vi "XY Plots from Image.vi"(10 "wavelengths":dbl[](array[numeric]), 11 "Image ROI1":u16[][](array[numeric])) -> (3 "Array":T1(array[cluster]))   [LabVIEW 2019, in "Dashboard.lvlib"]
uses:
  Dashboard.lvlib
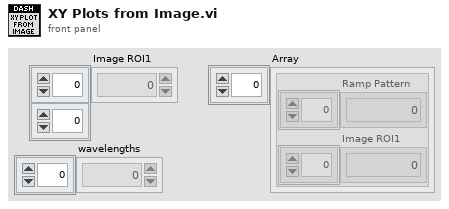
[diagram p1: front panel]
types:
  T1 = cluster{"Ramp Pattern":dbl[], "Image ROI1":u16[]}[]
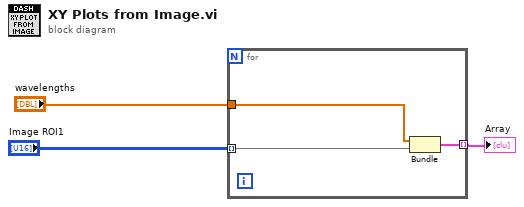
[diagram p0: block diagram]
diagram:
  n1 = for {
    tunnel: "Image ROI1" -> [w5] mode=indexing
    tunnel: [w6] -> w2 mode=indexing
    tunnel: "wavelengths" -> [w4]
    n2 = Bundle("wavelengths"=w4, "Image ROI1"=w5) -> (w6:cluster{"wavelengths":dbl[], "Image ROI1":u16[]})  [unwired: 1 in]
  }
  "Array" <- w2
